vi "ItemSymbol.vi"() -> ()   [LabVIEW 2011]
panel:
  in  "Listbox 2":i32(listbox)
  in  "Listbox":i32(listbox)
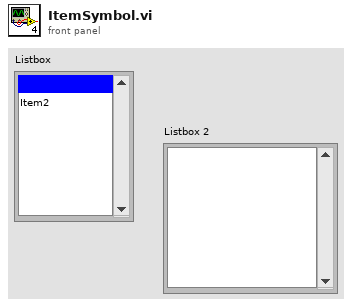
[diagram p1: front panel]
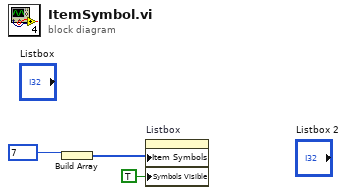
[diagram p0: block diagram]
diagram:
  n1 = Build Array(7) -> (w2:i32[])
  n2 = property on="Listbox" class="LstBox (strict)"("Item Symbols"=w2, "Symbols Visible"=TRUE ("Visible Items:Symbols Visible")) -> ()  [unwired: 2 in, 2 out]
